vi "TrapProfConstraint_New.vi"(9 "Max Accel":dbl format="%20.4f", 11 "Max Speed (M/S)":dbl format="%20.4f") -> (3 "TRAPEZOID_PROFILE_CONSTRAINT":T1 {"MaxAcceleration" format="%16_6e"; "MaxVelocity" format="%16_6e"})   [LabVIEW 2019, in "Trajectory_Library.lvlib"]
doc: "Construct constraint data cluster for a TrapezoidProfileConstraint\n \nInputs:\n - maxVelocity -- maximum velocity\n - maxAcceleration -- maximum acceleration\n\nOutputs:\n - Trapezoid_Profile_Constraint -- Updated Trapezoid_Profile_Constraint data cluster"
uses:
  Trajectory_Library.lvlib
  TypeDef/TRAPEZOID_PROFILE_CONSTRAINT.ctl
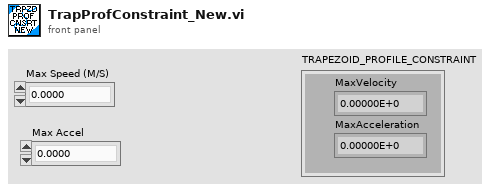
[diagram p1: front panel]
types:
  T1 = typedef "Trajectory_Library.lvlib/TRAPEZOID_PROFILE_CONSTRAINT.ctl" = cluster{"MaxVelocity":dbl, "MaxAcceleration":dbl}
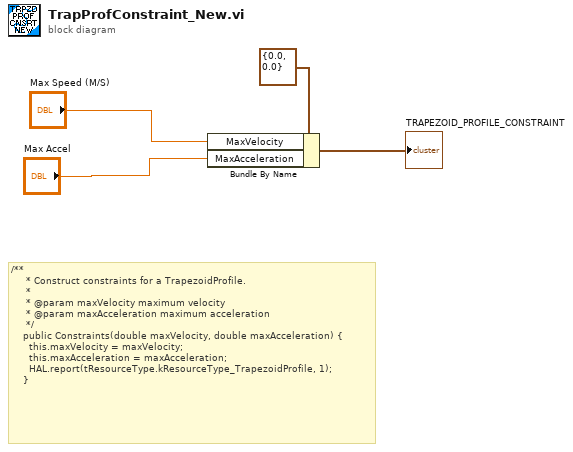
[diagram p0: block diagram]
diagram:
  # "/**\n     * Construct constraints for a TrapezoidProfile.\n     *\n     * @param maxVelocity maximum velocity\n     * @param maxAcceleration maximum acceleration\n     */\n    public Constraints(double maxVelocity, double maxAcceleration) {\n      this.maxVelocity = maxVelocity;\n      this.maxAcceleration = maxAcceleration;\n      HAL.report(tResourceType.kResourceType_TrapezoidProfile, 1);\n    }"
  n1 = Bundle By Name(cluster=T1 {"MaxVelocity"=0.0, "MaxAcceleration"=0.0} ("TRAPEZOID_PROFILE_CONSTRAINT"), "MaxVelocity"="Max Speed (M/S)", "MaxAcceleration"="Max Accel") -> (→"TRAPEZOID_PROFILE_CONSTRAINT":T1)
